vi "FlatToRichnixnet_grpc_SessionInfoResponse.vi"(5 "OutputClusterType":T1, 11 "InputCluster":T3) -> (3 "OutputCluster":T1)   [LabVIEW 2025, in "xnet-grpc_client.lvlib"]
uses:
  xnet-grpc_client.lvlib
  nixnet_grpc_SessionInfoResponse_Flat.ctl
  nixnet_grpc_SessionInfoState.ctl
  nixnet_grpc_SessionInfoResponse.ctl
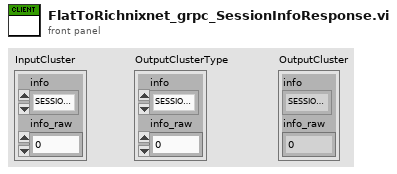
[diagram p1: front panel]
types:
  T1 = typedef "xnet-grpc_client.lvlib/nixnet_grpc_SessionInfoResponse.ctl" = cluster{"info":T2, "info_raw":u32}
  T2 = typedef "xnet-grpc_client.lvlib/nixnet_grpc_SessionInfoState.ctl" = enum32{"SESSION_INFO_STATE_STOPPED", "SESSION_INFO_STATE_STARTED", "SESSION_INFO_STATE_MIX"}
  T3 = typedef "xnet-grpc_client.lvlib/nixnet_grpc_SessionInfoResponse_Flat.ctl" = cluster{"info":T2, "info_raw":u32}
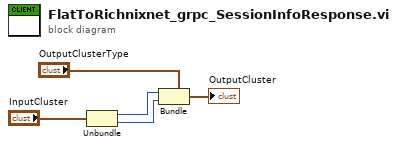
[diagram p0: block diagram]
diagram:
  n1 = Unbundle "Unbundle"("InputCluster") -> ("info"=w2:T2, "info_raw"=w1:u32)
  n2 = Bundle "Bundle"(cluster="OutputClusterType", "info"=w2, "info_raw"=w1) -> (→"OutputCluster":T1)
